vi "Unsupported Function.vi"(8 "error in":errorcluster, 10 "Function":string, 11 "PowerSupply in":refnum<class "PowerSupply.lvclass">) -> (0 "error out":errorcluster, 3 "PowerSupply out":refnum<class "PowerSupply.lvclass">)   [LabVIEW 2019, in "PowerSupply.lvlib" / "PowerSupply.lvclass"]
uses:
  Library/PowerSupply.lvclass
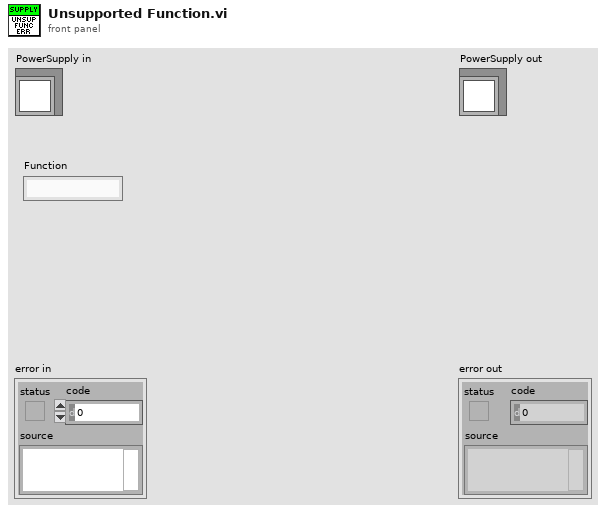
[diagram p1: front panel]
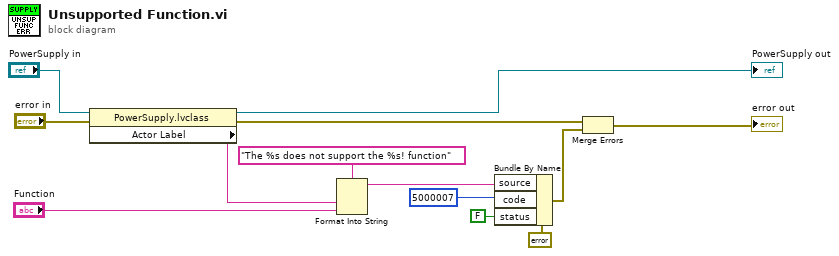
[diagram p0: block diagram]
diagram:
  n1 = property class="PowerSupply.lvclass"(reference="PowerSupply in", error in="error in") -> (reference out=→"PowerSupply out":refnum<class "PowerSupply.lvclass">, error out=w4:errorcluster, "Actor Label"=w12:string)
  n2 = Format Into String(format string="The %s does not support the %s! function", w12, "Function") -> (resulting string=w10:string)  [unwired: 2 in, 1 out]
  n3 = Bundle By Name(cluster=errorcluster {"status"=FALSE, "code"=0, "source"=""} ("output cluster"), "source"=w10, "code"=5000007, "status"=FALSE) -> (w11:errorcluster)
  n4 = Merge Errors(w4, w11) -> (→"error out":errorcluster)
